vi "Module Get.vi"(8 "error in (no error)":errorcluster, 11 "ID":i32) -> (0 "error out":errorcluster, 3 "Module":T1)   [LabVIEW 2022 SP3, in "Core.lvlib"]
uses:
  Core.lvlib
  Controls/Module.ctl
  Controls/Module Instance.ctl
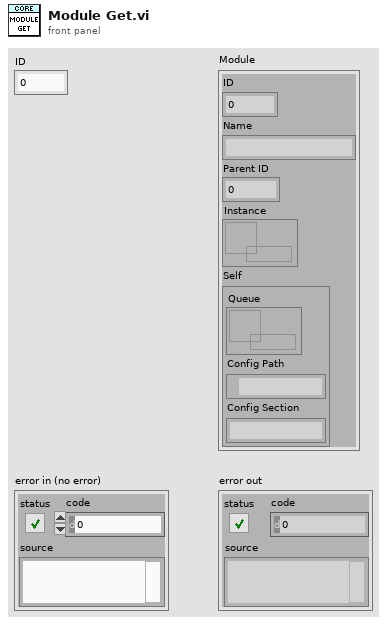
[diagram p1: front panel]
types:
  T1 = typedef "Core.lvlib/Module.ctl" = cluster{"ID":i32, "Name":string, "Parent ID":i32, "Instance":refnum<data-value>, "Self":T2}
  T2 = typedef "Core.lvlib/Module Instance.ctl" = cluster{"Queue":refnum<queue>, "Config Path":path, "Config Section":string}
  T3 = cluster{"ID":i32, "Name":string, "Parent ID":i32, "Instance":refnum<data-value>}[]
  T4 = cluster{"ID":i32, "Name":string, "Parent ID":i32, "Instance":refnum<data-value>}
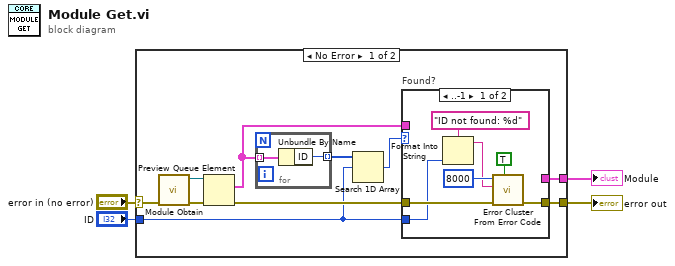
[diagram p0: block diagram]
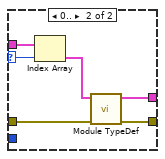
[diagram p2: hidden frame]
diagram:
  n1 = case shown="No Error" "error in (no error)" {
    selector: "error in (no error)" -> [w14 w30]
    tunnel: "ID" -> [w7 _]
    tunnel: [w10 w30] -> w2
    tunnel: [w9 _] -> w1
    frame No Error {
      n2 = call "Module Obtain.vi"("error in (no error)"=w14) -> ("error out"=w13:errorcluster, "Modules"=w6:refnum<queue>)  [unwired: 8 in, 1 out]
      n3 = Preview Queue Element(queue=w6, error in (no error)=w13) -> (element=w12:T3, error out=w11:errorcluster)  [unwired: 1 in, 2 out]
      n4 = for {
        tunnel: w12 -> [w16] mode=indexing
        tunnel: [w15] -> w5 mode=indexing
        n5 = Unbundle By Name(w16) -> ("ID"=w15:i32)
      }
      n6 = Search 1D Array(1D array=w5, element=w7) -> (index of element=w8:i32)  [unwired: 1 in]
      n7 = case "Found?" shown="..-1" w8 {
        selector: w8 -> [_ w24]
        tunnel: w12 -> [_ w29]
        tunnel: w11 -> [w23 w28]
        tunnel: [w22 w27] -> w10
        tunnel: [_ w25] -> w9
        tunnel: w7 -> [w19 _]
        frame ..-1 {
          n8 = Format Into String(format string="ID not found: %d", w19) -> (resulting string=w17:string)  [unwired: 2 in, 1 out]
          n9 = call <vilib>:"Error Cluster From Error Code.vi"("show call chain? (False)"=TRUE, "error in (no error)"=w23, "error message (\"\")"=w17, "error code (0)"=8000) -> ("error out"=w22:errorcluster)  [unwired: 5 in]
        }
        frame 0.. {
          n10 = Index Array(array=w29, index=w24) -> (element=w26:T4)
          n11 = call "Module TypeDef.vi"("error in (no error)"=w28, "Module in"=w26) -> ("error out"=w27:errorcluster, "Module"=w25:T1)  [unwired: 8 in]
        }
      }
    }
    frame Error {
    }
  }
  "error out" <- w2
  "Module" <- w1
